vi "String to Tree Preparation.vi"(1 "user formula":string, 2 "dummy":T2) -> (0 "empty structure":T1(array[cluster]))   [LabVIEW 2017, in "NI_Gmath.lvlib"]
uses:
  NI_Gmath.lvlib
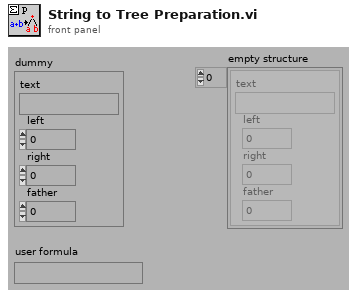
[diagram p1: front panel]
types:
  T1 = cluster{"text":string, "left":i32, "right":i32, "father":i32}[]
  T2 = cluster{"text":string, "left":i32, "right":i32, "father":i32}
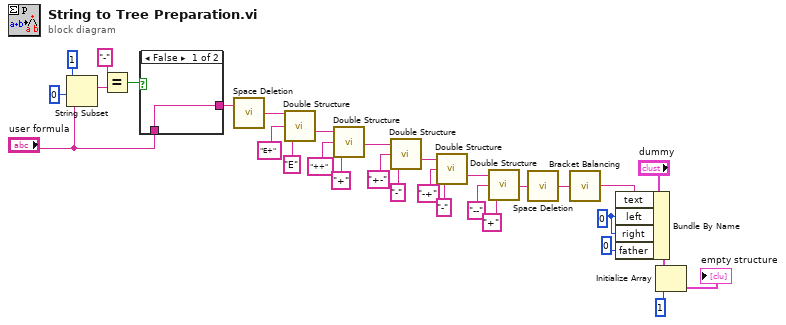
[diagram p0: block diagram]
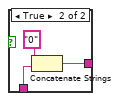
[diagram p2: hidden frame]
diagram:
  w2 = 0
  n1 = String Subset(string="user formula", offset (0)=0, length (rest)=1) -> (substring=w20:string)
  n2 = Equal?(x="-", y=w20) -> (x = y?=w22:bool)
  n3 = case shown="False" w22 {
    tunnel: "user formula" -> [w32 w35]
    tunnel: [w32 w34] -> w24
    frame False {
    }
    frame True {
      n4 = Concatenate Strings("0", w35) -> (w34:string)
    }
  }
  n5 = call "Space Deletion.vi"("string with spaces"=w24) -> ("string without spaces"=w30:string)
  n6 = call "Double Structure.vi"("change"="E", "-+ structure"="E+", "string"=w30) -> ("- structure"=w31:string)
  n7 = call "Double Structure.vi"("change"="+", "-+ structure"="++", "string"=w31) -> ("- structure"=w15:string)
  n8 = call "Double Structure.vi"("change"="-", "-+ structure"="+-", "string"=w15) -> ("- structure"=w16:string)
  n9 = call "Double Structure.vi"("change"="-", "-+ structure"="-+", "string"=w16) -> ("- structure"=w17:string)
  n10 = call "Double Structure.vi"("change"="+", "-+ structure"="--", "string"=w17) -> ("- structure"=w26:string)
  n11 = call "Space Deletion.vi"("string with spaces"=w26) -> ("string without spaces"=w27:string)
  n12 = call "Bracket Balancing.VI"("string before"=w27) -> ("string after"=w6:string)
  n13 = Bundle By Name(cluster="dummy", "text"=w6, "left"=w2, "right"=w2, "father"=0) -> (w4:T2)
  n14 = Initialize Array(w4, 1) -> (→"empty structure":T1)
